vi "Set Editor Mode.vi"(8 "Error In":errorcluster, 10 "Mode in":T1, 11 "Component.JSONEditor in":refnum<class "Component.JSONEditor.lvclass">) -> (0 "Error Out":errorcluster, 3 "Component.JSONEditor out":refnum<class "Component.JSONEditor.lvclass">)   [LabVIEW 2021, in "Component.JSONEditor.lvclass"]
uses:
  Component.JSONEditor.lvclass
  E:/Git/WebView-Components/Source/Component_class/Component.lvclass
  <vilib>/JDP Science/JSONtext/LVClass Serializer/JSONtext LVClass Serializer.lvclass
  <vilib>/sklein/WebView2/Webview2 Lib/WebView2 Control Object/WebView2 Control.lvclass
  f8653de4-75b8-4eba-bbea-61abc822b106.vi
  Editor Mode--enum.ctl
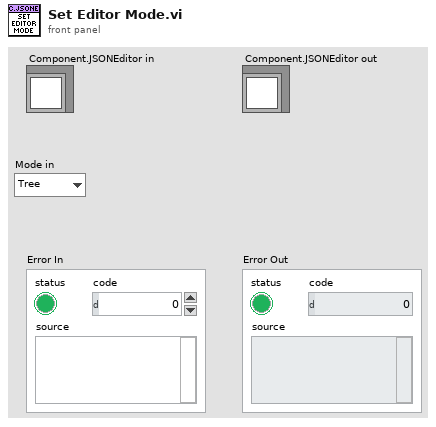
[diagram p1: front panel]
types:
  T1 = typedef "Component.JSONEditor.lvclass/Editor Mode--enum.ctl" = enum16{"Tree", "View", "Form", "Code", "Text"}
  T2 = cluster{"type":enum16{"loadJSON", "setMode", "getJSON"}, "mode":string}
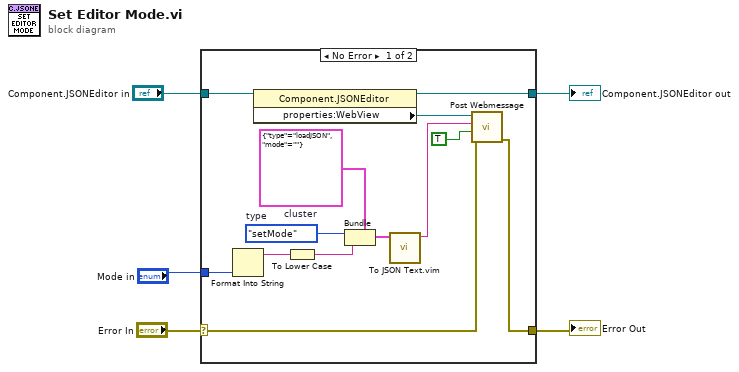
[diagram p0: block diagram]
diagram:
  n1 = case shown="No Error" "Error In" {
    selector: "Error In" -> [w8 w20]
    tunnel: [w7 w20] -> w4
    tunnel: [w9 w19] -> w2
    tunnel: "Component.JSONEditor in" -> [w16 w19]
    tunnel: "Mode in" -> [w18 _]
    frame No Error {
      w12 = T2 {"type"=enum."loadJSON", "mode"=""}  # cluster
      w15 = enum16{"loadJSON", "setMode", "getJSON"}."setMode"  # type
      n2 = Format Into String(w18) -> (resulting string=w17:string)  [unwired: 3 in, 1 out]
      n3 = property class="Component.JSONEditor"(reference=w16) -> (reference out=w9:refnum<class "Component.JSONEditor.lvclass">, "properties:WebView"=w10:refnum<class "WebView2 Control.lvclass">)  [unwired: 1 in, 1 out]
      n4 = To Lower Case(string=w17) -> (all lower case string=w14:string)
      n5 = Bundle(cluster=w12, "type"=w15, "mode"=w14) -> (w13:T2)
      n6 = call "To JSON Text.vim"("Anything"=w13) -> ("<JSON>"=w6:string)  [unwired: 9 in, 1 out]
      n7 = call <vilib>:"Post Webmessage.vi"("error in (no error)"=w8, "Send as JSON"=TRUE, "Message"=w6, "WebView2 Control in"=w10) -> ("error out"=w7:errorcluster)  [unwired: 6 in, 1 out]
    }
    frame Error {
    }
  }
  "Error Out" <- w4
  "Component.JSONEditor out" <- w2
